vi "Done.vi"(8 "error in (no error)":errorcluster, 11 "ConsoleSink in":refnum<class "ConsoleSink.lvclass">) -> (0 "error out":errorcluster)   [LabVIEW 2020, in "ConsoleView.lvlib" / "ConsoleSink.lvclass"]
doc: "--\nCopyright © 2017 Composed SystemsI All rights reserved.\n\nAuthor: Jon McBee <jon.mcbee@composed.io>\n\nThis library is provided \"AS IS\" ,WITHOUT WARRANTIES OR\nCONDITIONS OF ANY KIND, either express or implied.\n\nComposed Systems -- composed.io\n\nStream 0.0.1.1\nJon McBee - Composed Systems\nCopyright (c) 2017, Composed Systems"
uses:
  <vilib>/gpm_packages/@cs/event-logger/Source/ConsoleView/Sink/ConsoleSink.lvclass
  <vilib>/gpm_packages/@cs/event-logger/Source/ConsoleView/Sink/ConsoleSink.lvclass/ConsoleSink.ctl
  <vilib>/gpm_packages/@cs/event-logger/Source/Composed Log/Types/MessageCluster.ctl
  <vilib>/gpm_packages/@cs/event-logger/Source/Composed Log/Composed Log.lvlib
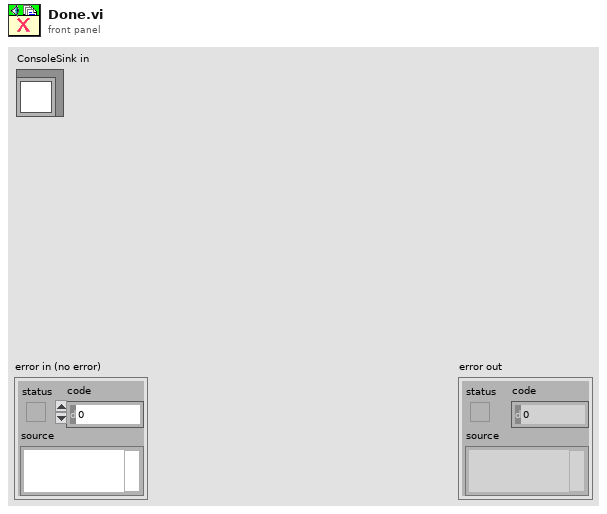
[diagram p1: front panel]
types:
  T1 = typedef "Composed Log.lvlib/MessageCluster.ctl" = cluster{"Message":string, "Data":variant}
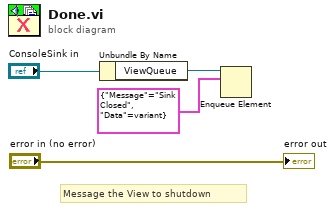
[diagram p0: block diagram]
diagram:
  # "Message the View to shutdown"
  n1 = Unbundle By Name("ConsoleSink in") -> ("ViewQueue"=w2:refnum<queue>)
  n2 = Enqueue Element(queue=w2, element=T1 {"Message"="Sink Closed", "Data"=variant}) -> ()  [unwired: 2 in, 3 out]
  "error out" <- "error in (no error)"
